vi "ZoneVacCtrldPickDrop.vi"(4 "Position":enum16{"1", "2"}(ring), 6 "Zone":enum16{"ZoneA", "ZoneB", "ZoneC", "ZoneD"}(ring), 7 "VacuumState":u8, 8 "error in (no error)":errorcluster, 9 "controller in":refnum<k24>, 10 "Zspeed":dbl=50.0 format="%#_13g", 11 "Z":dbl=65.0) -> (0 "error out":errorcluster, 3 "controller out":refnum<k24>)   [LabVIEW 2021]
uses:
  C:/Users/TTUHEP/Documents/LabVIEW/Other Models/2010/Bin/Aerotech.A3200.dll
  Other Models/2010/Bin/Aerotech.A3200.dll
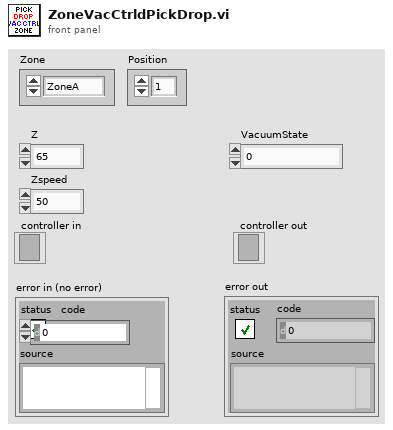
[diagram p1: front panel]
types:
  T1 = enum16{"BinarySwitch", "DecimalSwitch", "Conversion"}
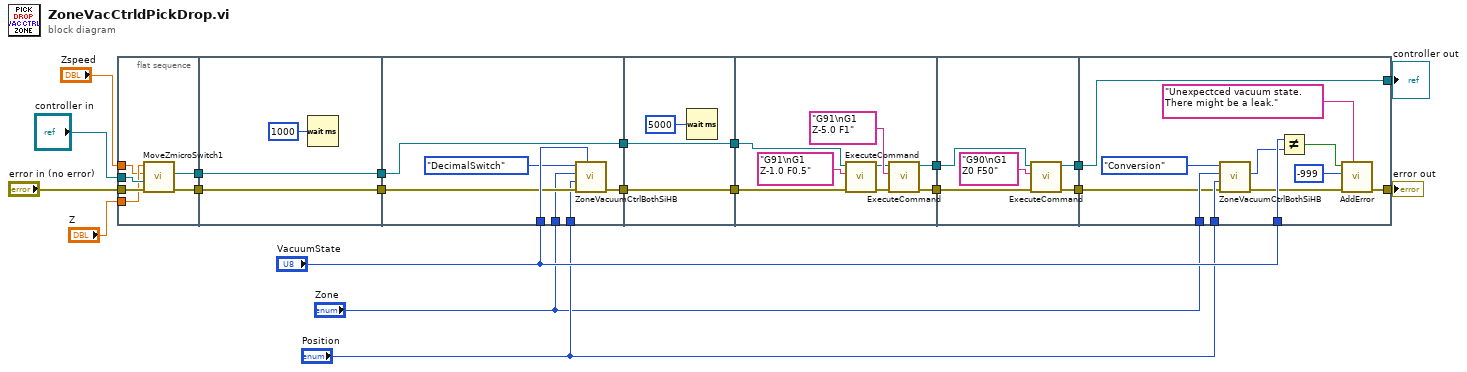
[diagram p0: block diagram]
diagram:
  n1 = flat-sequence {
    tunnel: [w24] -> w4
    tunnel: [w25] -> w2
    tunnel: "controller in" -> [w27]
    tunnel: "error in (no error)" -> [w26]
    tunnel: "Z" -> [w23]
    tunnel: "Zspeed" -> [w22]
    tunnel: w4 -> [w30]
    tunnel: [w30] -> w3
    tunnel: w2 -> [w29]
    tunnel: [w29] -> w1
    tunnel: w3 -> [w35]
    tunnel: [w32] -> w17
    tunnel: [w37] -> w16
    tunnel: w1 -> [w37]
    tunnel: "VacuumState" -> [w36]
    tunnel: "Position" -> [w34]
    tunnel: "Zone" -> [w33]
    tunnel: w17 -> [w40]
    tunnel: [w40] -> w12
    tunnel: w16 -> [w39]
    tunnel: [w39] -> w10
    tunnel: w12 -> [w46]
    tunnel: [w41] -> w11
    tunnel: w10 -> [w47]
    tunnel: [w42] -> w9
    tunnel: w11 -> [w53]
    tunnel: w9 -> [w51]
    tunnel: [w50] -> w15
    tunnel: [w49] -> w7
    tunnel: w15 -> [w62]
    tunnel: [w63] -> w14
    tunnel: [w62] -> w13
    tunnel: "VacuumState" -> [w61]
    tunnel: w7 -> [w57]
    tunnel: "Position" -> [w60]
    tunnel: "Zone" -> [w59]
    frame #0 {
      n2 = call "MoveZmicroSwitch1.vi"("Z"=w23, "Zspeed"=w22, "controller in"=w27, "error in (no error)"=w26) -> ("controller out"=w25:refnum<k24>, "error out"=w24:errorcluster)  [unwired: 3 in, 2 out]
    }
    frame #1 {
      n3 = Wait (ms)(milliseconds to wait=u32 1000) -> ()  [unwired: 1 out]
    }
    frame #2 {
      n4 = call "ZoneVacuumCtrlBothSiHB.vi"("DecimalIn"=w36, "Error In"=w35, "Position"=w34, "Zone"=w33, "ControlType"=T1."DecimalSwitch") -> ("Error Out"=w32:errorcluster)  [unwired: 4 in, 2 out]
    }
    frame #3 {
      n5 = Wait (ms)(milliseconds to wait=u32 5000) -> ()  [unwired: 1 out]
    }
    frame #4 {
      n6 = call "ExecuteCommand.vi"("error in (no error)"=w46, "Command Code"="G91\nG1 Z-1.0 F0.5", "controller in"=w47) -> ("error out"=w43:errorcluster, "controller out"=w44:refnum<k24>)  [unwired: 6 in, 1 out]
      n7 = call "ExecuteCommand.vi"("error in (no error)"=w43, "Command Code"="G91\nG1 Z-5.0 F1", "controller in"=w44) -> ("error out"=w41:errorcluster, "controller out"=w42:refnum<k24>)  [unwired: 6 in, 1 out]
    }
    frame #5 {
      n8 = call "ExecuteCommand.vi"("error in (no error)"=w53, "Command Code"="G90\nG1 Z0 F50", "controller in"=w51) -> ("error out"=w49:errorcluster, "controller out"=w50:refnum<k24>)  [unwired: 6 in, 1 out]
    }
    frame #6 {
      n9 = call "ZoneVacuumCtrlBothSiHB.vi"("Error In"=w57, "Position"=w60, "Zone"=w59, "ControlType"=T1."Conversion") -> ("Error Out"=w58:errorcluster, "DecimalOut"=w55:u32)  [unwired: 5 in, 1 out]
      n10 = Not Equal?(x=w61, y=w55) -> (x != y?=w54:bool)
      n11 = call "AddError.vi"("ErrorMessage"="Unexpectced vacuum state. There might be a leak.", "error in"=w58, "code"=-999, "Error?"=w54) -> ("Error out"=w63:errorcluster)  [unwired: 7 in]
    }
  }
  "controller out" <- w13
  "error out" <- w14
